vi "getRIOvalues.vi"(8 "error in":errorcluster, 11 "element":variant) -> (0 "error out":errorcluster, 1 "data":string[](array[string]), 2 "names":string[](array[string]))   [LabVIEW 2013]
doc: "Reads and unpacks the most recently sent value from the ocu writter on the rio. Returns the value as a flattened string, the name, and it's type"
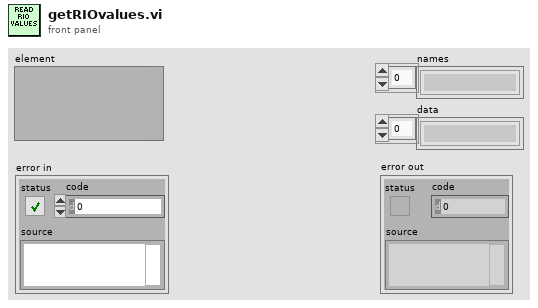
[diagram p1: front panel]
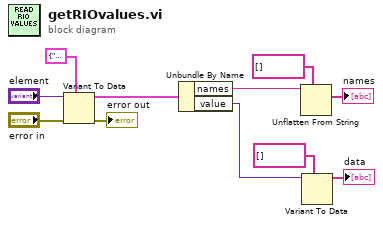
[diagram p0: block diagram]
diagram:
  n1 = Variant To Data(error in="error in", type=cluster{"names":string, "value":variant} {"names"="", "value"=variant} ("input cluster"), Variant="element") -> (data=w9:cluster{"names":string, "value":variant}, error out=→"error out":errorcluster)
  n2 = Unbundle By Name(w9) -> ("names"=w6:string, "value"=w4:variant)
  n3 = Unflatten From String(type=string[] [], binary string=w6) -> (value=→"names":string[])  [unwired: 3 in, 2 out]
  n4 = Variant To Data(type=string[] [], Variant=w4) -> (data=→"data":string[])  [unwired: 1 in, 1 out]
